vi "Initialize_SMU's.vi"(8 "Error In":errorcluster, 11 "Instrument_Visas":T1) -> (0 "Error Out":errorcluster)   [LabVIEW 2013]
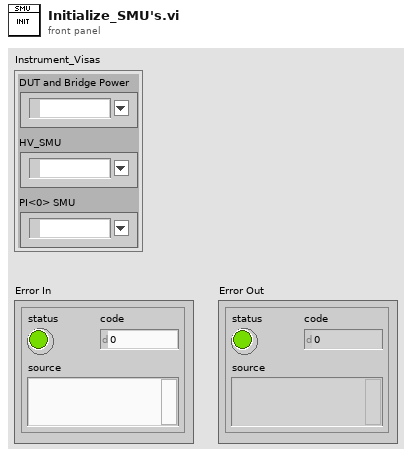
[diagram p1: front panel]
types:
  T1 = cluster{"DUT and Bridge Power":refnum<k15>, "HV_SMU":refnum<k15>, "PI<0> SMU":refnum<k15>}
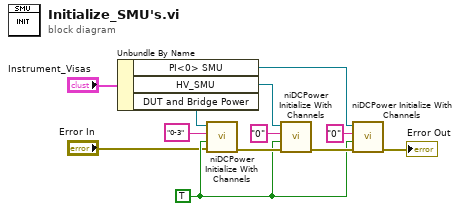
[diagram p0: block diagram]
diagram:
  w3 = TRUE ("reset (false)")
  n1 = Unbundle By Name("Instrument_Visas") -> ("PI<0> SMU"=w5:refnum<k15>, "HV_SMU"=w8:refnum<k15>, "DUT and Bridge Power"=w9:refnum<k15>)
  n2 = call <instrlib>:"niDCPower Initialize With Channels.vi"("error in (no error)"="Error In", "reset (false)"=w3, "channels"="0-3", "resource name"=w9) -> ("error out"=w11:errorcluster)  [unwired: 6 in, 1 out]
  n3 = call <instrlib>:"niDCPower Initialize With Channels.vi"("error in (no error)"=w11, "reset (false)"=w3, "channels"="0", "resource name"=w8) -> ("error out"=w10:errorcluster)  [unwired: 6 in, 1 out]
  n4 = call <instrlib>:"niDCPower Initialize With Channels.vi"("error in (no error)"=w10, "reset (false)"=w3, "channels"="0", "resource name"=w5) -> ("error out"=→"Error Out":errorcluster)  [unwired: 6 in, 1 out]
